vi "TDMSReadWriteTraces.vi"(6 "Data in":dbl[][](array[numeric]), 7 "Task":T1(ring), 8 "error in (no error)":errorcluster, 9 "Channels in":string[](array[string]), 10 "group name":string="None", 11 "tracename":string="E:\\users\\noort\\data\\270404\\_001.log") -> (0 "error out":errorcluster, 1 "Channels out":string[](array[string]), 2 "Group names out":string[](array[string]), 3 "tracename out":string="E:\\current VIs\\Vi\\Data\\data_074.tdms: 20", 4 "Data out":dbl[][](array[numeric]), 5 "size(s)":i32[](array[numeric]))   [LabVIEW 2018]
uses:
  <vilib>/Platform/storage/lvStorage.llb/_openStorageWithRootAutoDetect.vi
  <vilib>/Platform/storage/lvStorage.llb/xStorage/xStorageSupp/ErrorOut.vi
  <vilib>/Platform/storage/Storage.llb/__loadPropString.vi
  <vilib>/Platform/storage/Storage.llb/__loadPropTime.vi
  <vilib>/Platform/storage/Storage.llb/__loadPropRefList.vi
  <vilib>/Platform/storage/lvStorage.llb/_loadDDT.vi
  <vilib>/Platform/storage/Storage.llb/__loadPropFloat64.vi
  <vilib>/Platform/storage/lvStorage.llb/Delete Channel.vi
  <vilib>/Platform/storage/Storage.llb/Get Object Info.vi
  <vilib>/Platform/storage/Storage.llb/__closeStorageFromObject.vi
  <vilib>/Platform/storage/lvStorage.llb/xStorage/Open Data Storage/Open Data Storage.xnode
  <vilib>/Platform/storage/lvStorage.llb/xStorage/Get Properties/Get Properties.xnode
  <vilib>/Platform/storage/lvStorage.llb/xStorage/Close Data Storage/Close Data Storage.xnode
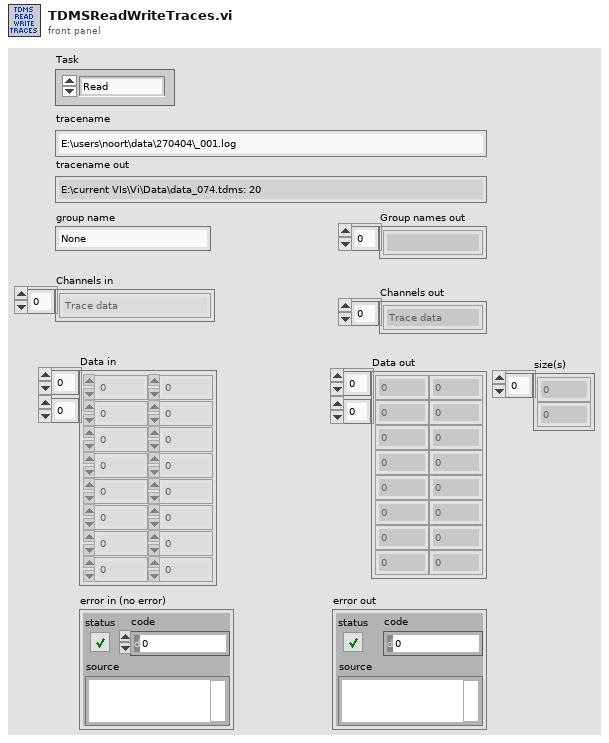
[diagram p1: front panel]
types:
  T1 = enum16{"Read", "Write", "Get channels", "Delete channels"}
  T2 = enum16{"open", "open or create", "create or replace", "create", "open (read-only)"}
  T3 = enum16{"open", "open or create", "create or replace", "create", "open (read only)"}
  T4 = enum16{"UPDATE", "READ", "QUERY", "CREATE CHILD", "CREATE", "CONNECT", "DISCONNECT"}
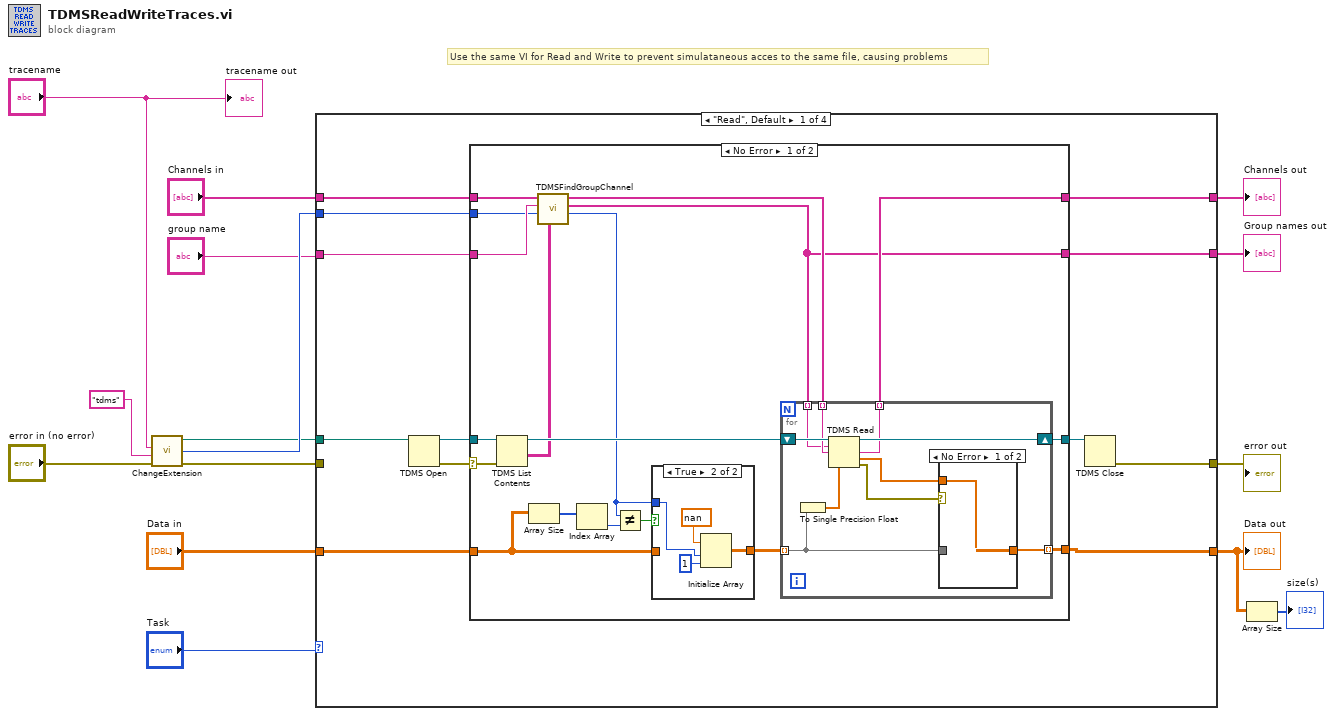
[diagram p0: block diagram]
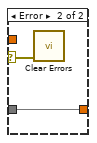
[diagram p3: hidden frame]
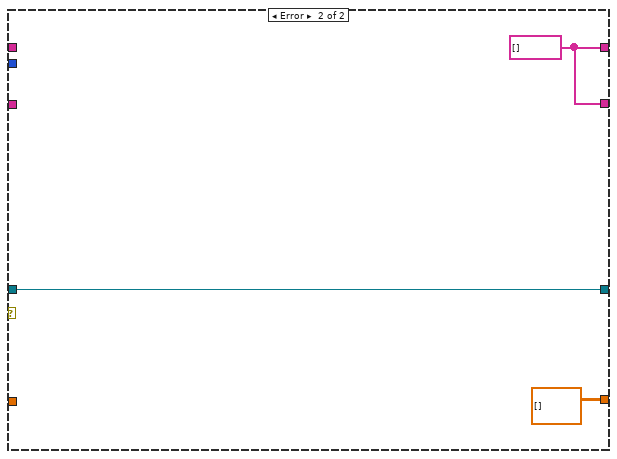
[diagram p4: hidden frame]
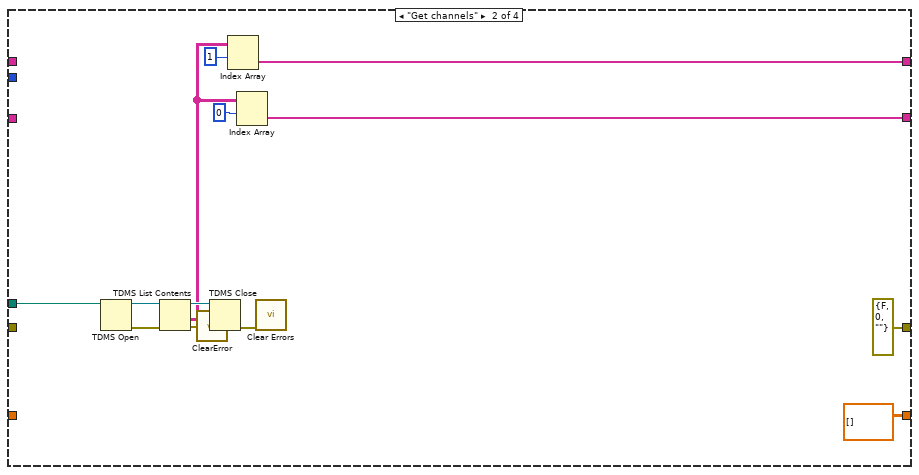
[diagram p5: hidden frame]
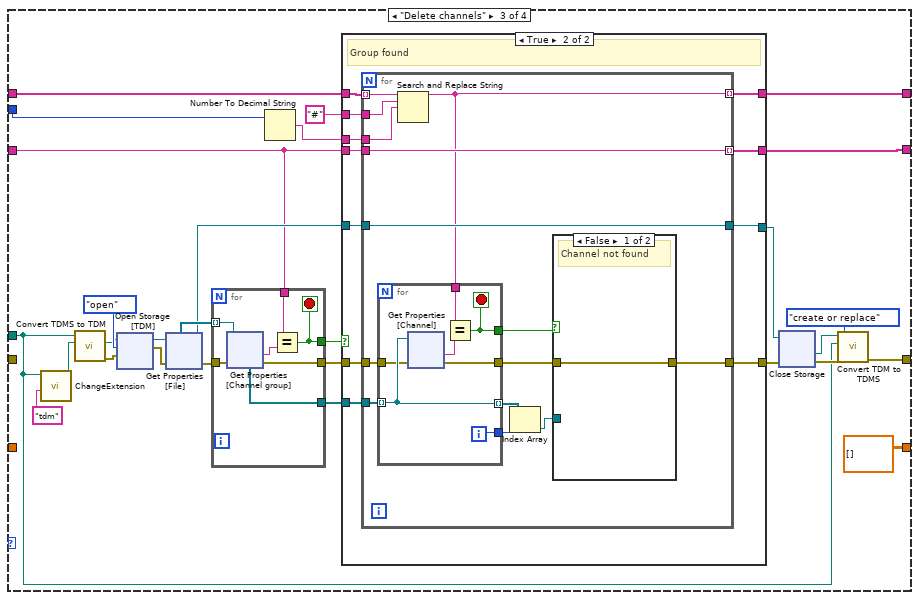
[diagram p6: hidden frame]
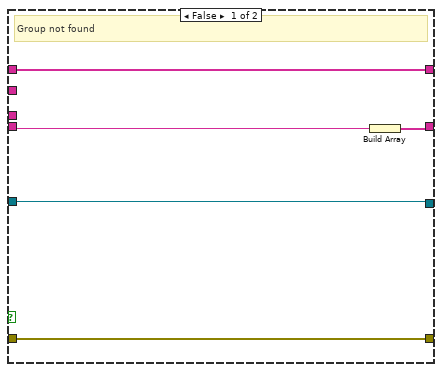
[diagram p7: hidden frame]
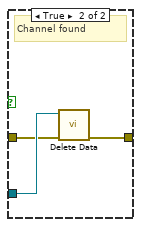
[diagram p8: hidden frame]
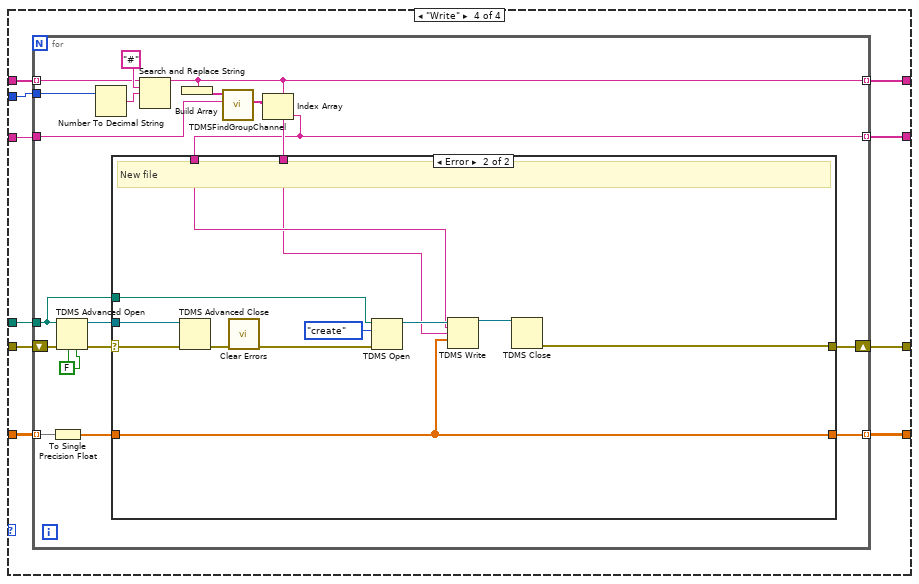
[diagram p9: hidden frame]
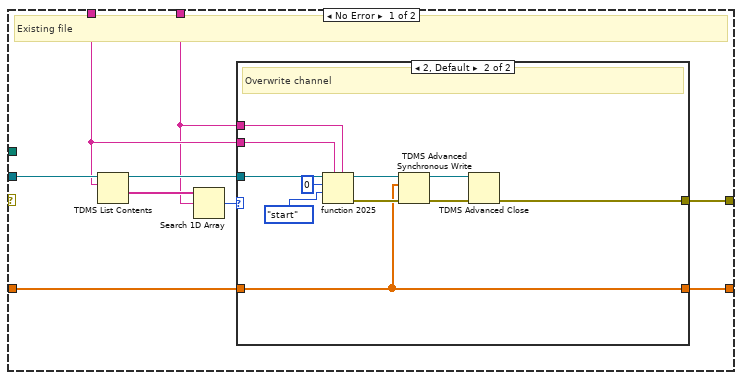
[diagram p10: hidden frame]
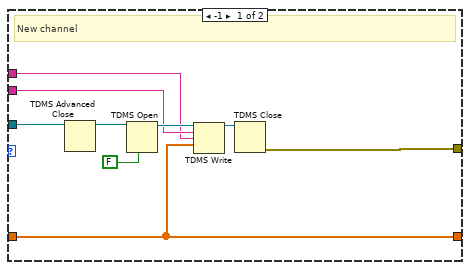
[diagram p11: hidden frame]
diagram:
  # "Use the same VI for Read and Write to prevent simulataneous acces to the same file, causing problems"
  n1 = call "ChangeExtension.vi"("error in (no error)"="error in (no error)", "extension"="tdms", "file in"="tracename") -> ("error out"=w8:errorcluster, "Path out"=w11:path, "Tracenr"=w14:i32)  [unwired: 2 in, 2 out]
  n2 = case shown="\"Read\", Default" "Task" {
    tunnel: "Data in" -> [w23 _ _ w255]
    tunnel: w14 -> [w20 _ w83 w254]
    tunnel: "Channels in" -> [w18 _ w98 w253]
    tunnel: "group name" -> [w19 _ w86 w252]
    tunnel: w11 -> [w24 w78 w92 w251]
    tunnel: [w21 errorcluster {"status"=FALSE, "code"=0, "source"=""} ("error out") w84 w250] -> w10
    tunnel: w8 -> [_ _ _ w249]
    tunnel: [w17 w76 w88 w248] -> w6
    tunnel: [w22 dbl[][] [] ("Data in") dbl[][] [] ("Data in") w247] -> w2
    tunnel: [w16 w73 w87 w246] -> w3
    frame "Read", Default {
      n3 = TDMS Open(11:w24) -> (0:w26:errorcluster, 3:w25:refnum<k34>)  [unwired: 6 in]
      n4 = case shown="No Error" w26 {
        selector: w26 -> [w43 _]
        tunnel: w25 -> [w45 w65]
        tunnel: w19 -> [w39 _]
        tunnel: [w40 dbl[][] []] -> w22
        tunnel: w20 -> [w37 _]
        tunnel: [w42 w65] -> w27
        tunnel: w23 -> [w29 _]
        tunnel: w18 -> [w36 _]
        tunnel: [w35 w64] -> w17
        tunnel: [w34 w64] -> w16
        frame No Error {
          n5 = TDMS List Contents(4:w43, 7:w45) -> (1:w38:string[][], 3:w44:refnum<k34>)  [unwired: 1 in, 2 out]
          n6 = Array Size(array=w29) -> (size(s)=w33:i32[])
          n7 = call "TDMSFindGroupChannel.vi"("groups/channels in file"=w38, "Tracenr"=w37, "Group in"=w39, "channels in"=w36) -> ("#Channels"=w28:i32, "Groups out"=w34:string[], "Channels out"=w41:string[])  [unwired: 3 in]
          n8 = Index Array(array=w33) -> (element=w32:i32)  [unwired: 1 in]
          n9 = Not Equal?(x=w28, y=w32) -> (x != y?=w31:bool)
          n10 = case shown="True" w31 {
            tunnel: [w46 w47] -> w30
            tunnel: w29 -> [w46 _]
            tunnel: w28 -> [_ w50]
            frame False {
            }
            frame True {
              n11 = Initialize Array(nan ("element"), w50, 1 ("dimension size")) -> (w47:dbl[][])
            }
          }
          n12 = for {
            tunnel: [w52] -> w35 mode=indexing
            tunnel: w30 -> [w53] mode=indexing
            tunnel: w41 -> [w58] mode=indexing
            shift-right: [w59] -> w42
            shift-left: w44 -> [w60]
            tunnel: w34 -> [w57] mode=indexing
            tunnel: [w55] -> w40 mode=indexing
            n13 = To Single Precision Float(number=w53) -> (single precision float=w51:sgl[])
            n14 = TDMS Read(0:w60, 5:w57, 7:w58, 12:w51) -> (4:w59:refnum<k34>, 8:w52:string, 10:w54:sgl[], 15:w56:errorcluster)  [unwired: 4 in, 2 out]
            n15 = case shown="No Error" w56 {
              selector: w56 -> [_ w62]
              tunnel: [w61 w63] -> w55
              tunnel: w54 -> [w61 _]
              tunnel: w53 -> [_ w63]
              frame No Error {
              }
              frame Error {
                n16 = call <vilib>:"Clear Errors.vi"("error in (no error)"=w62) -> ()  [unwired: 5 in, 2 out]
              }
            }
          }
        }
        frame Error {
          w64 = string[] []
        }
      }
      n17 = TDMS Close(11:w27) -> (0:w21:errorcluster)  [unwired: 1 in, 1 out]
    }
    frame "Get channels" {
      n18 = TDMS Open(11:w78) -> (0:w71:errorcluster, 3:w80:refnum<k34>)  [unwired: 6 in]
      n19 = TDMS List Contents(4:w71, 7:w80) -> (0:w67:errorcluster, 1:w75:string[][], 3:w79:refnum<k34>)  [unwired: 1 in, 1 out]
      n20 = call <vilib>:"ClearError.vi"("error in (no error)"=w67) -> ("error out"=w70:errorcluster)
      n21 = TDMS Close(8:w70, 11:w79) -> (0:w72:errorcluster)  [unwired: 1 out]
      n22 = Index Array(array=w75, index (row)=1) -> (element=w76:string[])  [unwired: 1 in]
      n23 = Index Array(array=w75, index (row)=0) -> (element=w73:string[])  [unwired: 1 in]
      n24 = call <vilib>:"Clear Errors.vi"("error in (no error)"=w72) -> ()  [unwired: 5 in, 2 out]
    }
    frame "Delete channels" {
      n25 = call "ChangeExtension.vi"("extension"="tdm", "Path in"=w92) -> ("Path out"=w107:path)  [unwired: 3 in, 4 out]
      n26 = call <vilib>:"Convert TDMS to TDM.vi"("target file path (*.tdm)"=w107, "source file path (*.tdms)"=w92) -> ("error out"=w89:errorcluster, "target file path (*.tdm) out"=w103:path)  [unwired: 2 in, 6 out]
      n27 = xnode ("Open Storage\n[TDM]")("file path"=w103, "function (open:0)"=T3."open" ("fonction (open : 0)"), "error in (no error)"=w89) -> ("storage refnum (file)"=w105:refnum<k20>, "error out"=w104:errorcluster)  [unwired: 2 in, 1 out]
      n28 = xnode ("Get Properties\n[File]")("storage refnum (file)"=w105, "error in"=w104) -> ("storage refnum (file) out"=w97:refnum<k20>, "error out"=w102:errorcluster, "storage refnums (channel group)"=w101:refnum<k20>[])  [unwired: 5 out]
      n29 = for {
        tunnel: w101 -> [w190] mode=indexing
        tunnel: w86 -> [w191]
        tunnel: w102 -> [w189]
        tunnel: [w188] -> w100
        tunnel: [w186] -> w99
        tunnel: [w185] -> w90
        stop <- w188 stop-if-true
        n30 = xnode ("Get Properties\n[Channel group]")("storage refnum (channel group)"=w190, "error in"=w189) -> ("error out"=w185:errorcluster, "Name"=w187:string, "storage refnums (channel)"=w186:refnum<k20>[])  [unwired: 2 out]
        n31 = Equal?(x=w191, y=w187) -> (x = y?=w188:bool)
      }
      n32 = Number To Decimal String(number=w83) -> (decimal integer string=w81:string)  [unwired: 1 in]
      n33 = case shown="True" w100 {
        tunnel: w99 -> [_ w132]
        tunnel: w98 -> [w119 w131]
        tunnel: [w121 w130] -> w96
        tunnel: w97 -> [w121 w129]
        tunnel: [w120 w128] -> w91
        tunnel: w90 -> [w120 w127]
        tunnel: [w119 w126] -> w88
        tunnel: [w117 w125] -> w87
        tunnel: w86 -> [w118 w124]
        tunnel: "#" ("substring (\"\")") -> [_ w123]
        tunnel: w81 -> [_ w122]
        frame False {
          # "Group not found"
          n34 = Build Array(w118) -> (w117:string[])
        }
        frame True {
          # "Group found"
          n35 = for {
            tunnel: w132 -> [w146]
            tunnel: w131 -> [w134] mode=indexing
            tunnel: [w141] -> w130
            tunnel: w129 -> [w141]
            tunnel: [w140] -> w128
            tunnel: w127 -> [w138]
            tunnel: [w133] -> w126 mode=indexing
            tunnel: [w137] -> w125 mode=indexing
            tunnel: w124 -> [w137]
            tunnel: w123 -> [w136]
            tunnel: w122 -> [w135]
            n36 = Search and Replace String(input string=w134, search string=w136, replace string=w135) -> (result string=w133:string)  [unwired: 5 in, 3 out]
            n37 = for {
              tunnel: w146 -> [w153] mode=indexing
              tunnel: w133 -> [w154]
              tunnel: [w157] -> w145
              tunnel: [w156] -> w142
              tunnel: [w153] -> w144 mode=indexing
              tunnel: [w152] -> w139
              tunnel: w138 -> [w151]
              i -> [w157]
              stop <- w156 stop-if-true
              n38 = xnode ("Get Properties\n[Channel]")("storage refnum (channel)"=w153, "error in"=w151) -> ("error out"=w152:errorcluster, "Name"=w155:string)  [unwired: 8 out]
              n39 = Equal?(x=w154, y=w155) -> (x = y?=w156:bool)
            }
            n40 = Index Array(array=w144, index=w145) -> (element=w143:refnum<k20>)
            n41 = case shown="False" w142 {
              tunnel: w143 -> [_ w150]
              tunnel: [w147 w149] -> w140
              tunnel: w139 -> [w147 w148]
              frame False {
                # "Channel not found"
              }
              frame True {
                # "Channel found"
                n42 = call-poly <vilib>:"Delete Data.vi"("error in (no error)"=w148, "storage refnum (channel)"=w150) -> ("error out"=w149:errorcluster)  [unwired: 5 out]
              }
            }
          }
        }
      }
      n43 = xnode ("Close Storage")("storage refnum (file)"=w96, "error in (no error)"=w91) -> ("file path"=w93:path, "error out"=w94:errorcluster)
      n44 = call <vilib>:"Convert TDM to TDMS.vi"("error in (no error)"=w94, "target file operation (2:create or replace)"=T2."create or replace", "target file path (*.tdms)"=w92, "source file path (*.tdm)"=w93) -> ("error out"=w84:errorcluster)  [unwired: 7 out]
    }
    frame "Write" {
      n45 = for {
        tunnel: w255 -> [w264] mode=indexing
        tunnel: w254 -> [w272]
        tunnel: w252 -> [w262]
        tunnel: w251 -> [w256]
        shift-right: [w267] -> w250
        shift-left: w249 -> [w266]
        tunnel: w253 -> [w270] mode=indexing
        tunnel: [w261] -> w248 mode=indexing
        tunnel: [w265] -> w247 mode=indexing
        tunnel: [w258] -> w246 mode=indexing
        w257 = FALSE ("disable buffering? (T)")
        n46 = To Single Precision Float(number=w264) -> (single precision float=w263:sgl[])
        n47 = TDMS Advanced Open(4:w257, 6:w257, 8:w266, 11:w256) -> (0:w269:errorcluster, 3:w268:refnum<k34>)  [unwired: 1 in, 1 out]
        n48 = Number To Decimal String(number=w272) -> (decimal integer string=w271:string)  [unwired: 1 in]
        n49 = Search and Replace String(input string=w270, search string="#", replace string=w271) -> (result string=w261:string)  [unwired: 5 in, 3 out]
        n50 = Build Array(w261) -> (w260:string[])
        n51 = call "TDMSFindGroupChannel.vi"("Group in"=w262, "channels in"=w260) -> ("Groups out"=w259:string[])  [unwired: 5 in, 2 out]
        n52 = Index Array(array=w259) -> (element=w258:string)  [unwired: 1 in]
        n53 = case shown="Error" w269 {
          selector: w269 -> [_ w313]
          tunnel: w263 -> [w282 w307]
          tunnel: w268 -> [w281 w314]
          tunnel: [w277 w309] -> w267
          tunnel: w258 -> [w275 w310]
          tunnel: w261 -> [w274 w308]
          tunnel: [w276 w307] -> w265
          tunnel: w256 -> [_ w303]
          frame No Error {
            # "Existing file"
            n54 = TDMS List Contents(6:w275, 7:w281) -> (1:w279:string[], 3:w280:refnum<k34>)  [unwired: 1 in, 2 out]
            n55 = Search 1D Array(1D array=w279, element=w274) -> (index of element=w278:i32)  [unwired: 1 in]
            n56 = case shown="2, Default" w278 {
              tunnel: w282 -> [w284 w292]
              tunnel: w280 -> [w290 w298]
              tunnel: [w287 w293] -> w277
              tunnel: [w284 w292] -> w276
              tunnel: w275 -> [w286 w297]
              tunnel: w274 -> [w285 w296]
              frame -1 {
                # "New channel"
                n57 = TDMS Advanced Close(11:w290) -> (3:w291:path)  [unwired: 3 in, 1 out]
                n58 = TDMS Open(6:FALSE ("disable buffering? (T)"), 11:w291) -> (3:w289:refnum<k34>)  [unwired: 5 in, 1 out]
                n59 = TDMS Write(0:w289, 5:w286, 7:w285, 9:w284) -> (4:w288:refnum<k34>)  [unwired: 2 in, 3 out]
                n60 = TDMS Close(11:w288) -> (0:w287:errorcluster)  [unwired: 1 in, 1 out]
              }
              frame 2, Default {
                # "Overwrite channel"
                n61 = fn#2025(5:w296, 7:w297, 9:enum16{"start", "end"}."start" ("from (0:start)"), 10:i64 0 ("offset (0)"), 11:w298) -> (0:w300:errorcluster, 3:w299:refnum<k34>)  [unwired: 1 in]
                n62 = TDMS Advanced Synchronous Write(8:w300, 10:w292, 11:w299) -> (0:w301:errorcluster, 3:w302:refnum<k34>)
                n63 = TDMS Advanced Close(8:w301, 11:w302) -> (0:w293:errorcluster)  [unwired: 2 in, 1 out]
              }
            }
          }
          frame Error {
            # "New file"
            n64 = TDMS Advanced Close(8:w313, 11:w314) -> (0:w306:errorcluster)  [unwired: 2 in, 1 out]
            n65 = call <vilib>:"Clear Errors.vi"("error in (no error)"=w306) -> ("error out"=w304:errorcluster)  [unwired: 5 in, 1 out]
            n66 = TDMS Open(8:w304, 10:T2."create" ("operation (0:open)"), 11:w303) -> (3:w312:refnum<k34>)  [unwired: 4 in, 1 out]
            n67 = TDMS Write(0:w312, 5:w310, 7:w308, 9:w307) -> (4:w311:refnum<k34>)  [unwired: 2 in, 3 out]
            n68 = TDMS Close(11:w311) -> (0:w309:errorcluster)  [unwired: 1 in, 1 out]
          }
        }
      }
    }
  }
  "error out" <- w10
  "Channels out" <- w6
  "Data out" <- w2
  "Group names out" <- w3
  n69 = Array Size(array=w2) -> (size(s)=→"size(s)":i32[])
  "tracename out" <- "tracename"
